vi "EA Calculations.vi"(10 "AC":dbl, 11 "DC":dbl) -> (3 "EA":dbl)   [LabVIEW 2017, in "Lockin and Keithley Multimeter.lvclass"]
uses:
  Lockin and Keithley Multimeter.lvclass
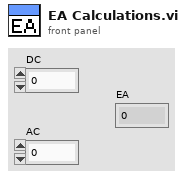
[diagram p1: front panel]
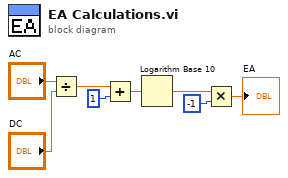
[diagram p0: block diagram]
diagram:
  n1 = Divide(x="AC", y="DC") -> (x/y=w6:dbl)
  n2 = Add(x=w6, y=1) -> (x+y=w1:dbl)
  n3 = Logarithm Base 10(1:w1) -> (0:w5:dbl)
  n4 = Multiply(x=w5, y=-1) -> (x*y=→"EA":dbl)
